vi "Perform measurements.vi"(6 "Measurement configuration":T2={"Number of channels to measure"=0, "Full scale range"=10.0, "Analog source input channels"=[], "Analog source resource names"=[], "Frequency"=1000.0, "Amplitude"=-1.0, "Digital capture resource name"="", "Digital capture sample rate"=800000.0, "Digital capture samples"=800000}, 10 "DPI Session":refnum<k15>, 11 "DPI Bitfile reference":refnum<k20>) -> (0 "error out":errorcluster, 2 "Measurement results":T1)   [LabVIEW 2021, in "adc_acMultiChannelMeasurement.lvlib"]
uses:
  adc_acMultiChannelMeasurement.lvlib
  Measurement Configuration.ctl
  Measurement Results.ctl
  <vilib>/Utility/error.llb/Error Cluster From Error Code.vi
  <vilib>/rvi/errors/niLvFpgaAdjustHostInterfaceError.vi
  <instrlib>/niDigital/niDigital.llb/niDigital Burst Pattern (Burst Only).vi
  <vilib>/rvi/interface/nirviReadWriteControl/nirviReadWriteControl.xnode
  NiFpgaLv.dll
  <vilib>/rvi/interface/Simulation/niFpgaSimulationCallBeginRW.vi
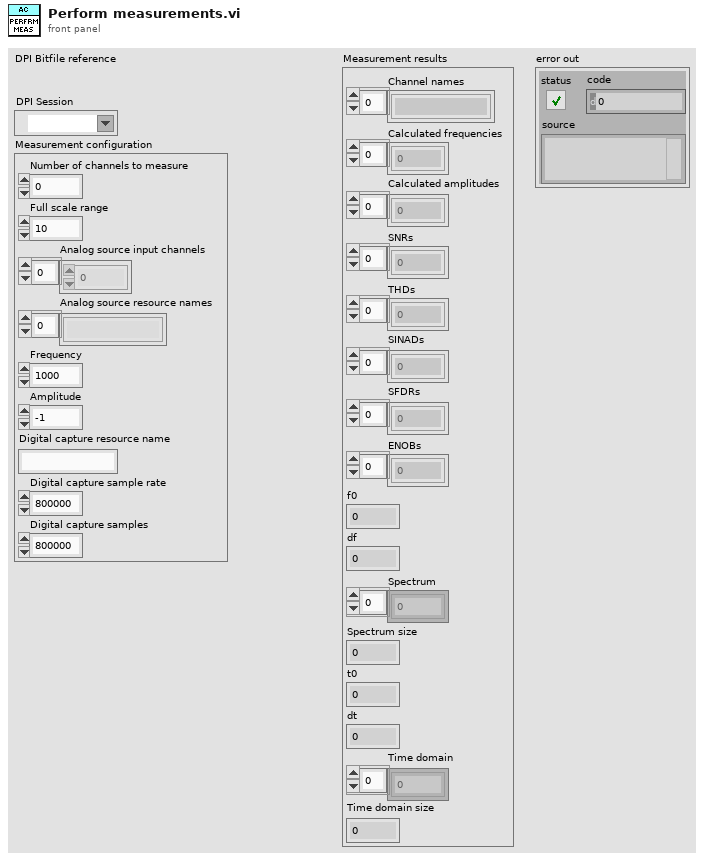
[diagram p1: front panel]
types:
  T1 = typedef "adc_acMultiChannelMeasurement.lvlib/Measurement Results.ctl" = cluster{"Channel names":string[], "Calculated frequencies":dbl[], "Calculated amplitudes":dbl[], "SNRs":dbl[], "THDs":dbl[], "SINADs":dbl[], "SFDRs":dbl[], "ENOBs":dbl[], "f0":dbl, "df":dbl, "Spectrum":dbl[], "Spectrum size":i32, "t0":dbl, "dt":dbl, "Time domain":dbl[], "Time domain size":i32}
  T2 = typedef "adc_acMultiChannelMeasurement.lvlib/Measurement Configuration.ctl" = cluster{"Number of channels to measure":i32, "Full scale range":dbl, "Analog source input channels":i32[], "Analog source resource names":string[], "Frequency":dbl, "Amplitude":dbl, "Digital capture resource name":string, "Digital capture sample rate":dbl, "Digital capture samples":u32}
  T3 = cluster{"Detected frequency":dbl, "Detected amplitude":dbl, "SNR":dbl, "THD":dbl, "SINAD":dbl, "SFDR":dbl, "ENOB":dbl}
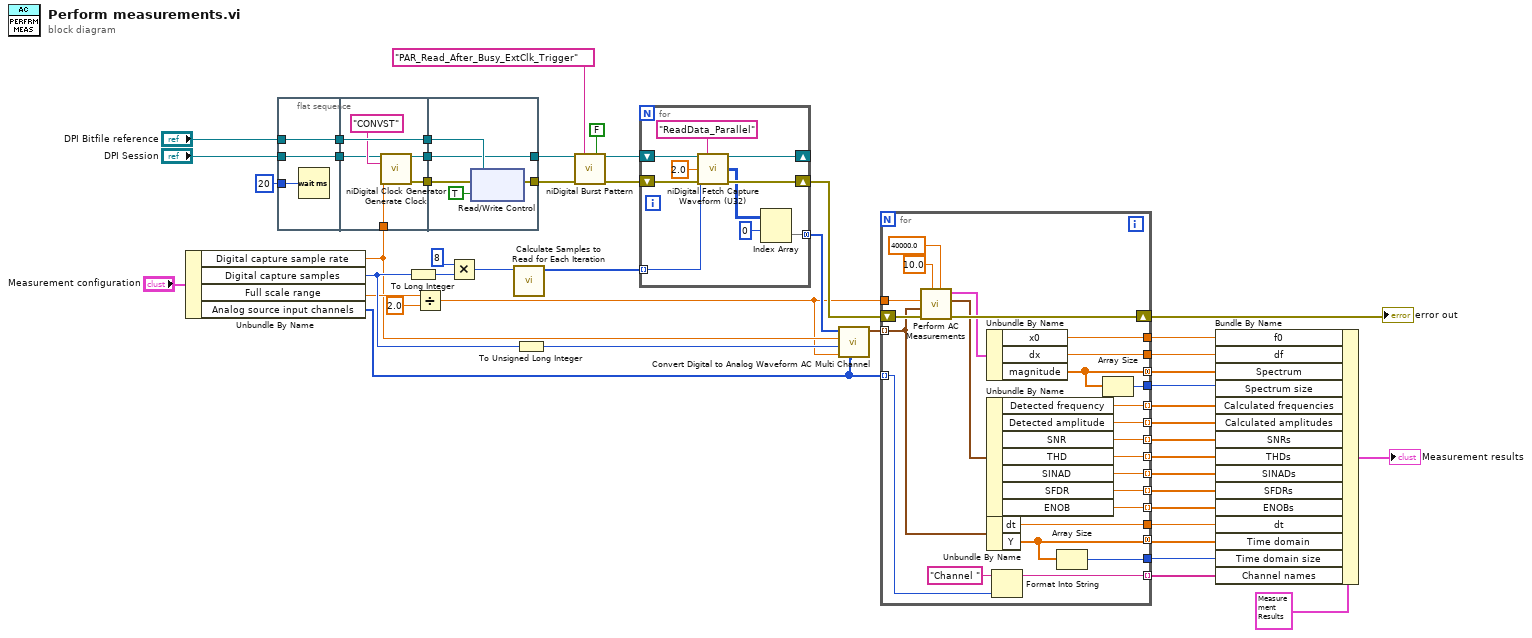
[diagram p0: block diagram]
diagram:
  n1 = Unbundle By Name("Measurement configuration") -> ("Digital capture sample rate"=w8:dbl, "Digital capture samples"=w13:u32, "Full scale range"=w10:dbl, "Analog source input channels"=w1:i32[])
  n2 = flat-sequence {
    tunnel: "DPI Session" -> [w49]
    tunnel: "DPI Bitfile reference" -> [w50]
    tunnel: [w50] -> w35
    tunnel: [w49] -> w34
    tunnel: u32 20 ("milliseconds to wait") -> [w48]
    tunnel: [w56] -> w33
    tunnel: [w54] -> w32
    tunnel: [w52] -> w31
    tunnel: w8 -> [w51]
    tunnel: w35 -> [w56]
    tunnel: w34 -> [w53]
    tunnel: [w61] -> w47
    tunnel: w33 -> [w60]
    tunnel: w32 -> [w58]
    tunnel: [w57] -> w36
    tunnel: w31 -> [w57]
    frame #0 {
      n3 = Wait (ms)(milliseconds to wait=w48) -> ()  [unwired: 1 out]
    }
    frame #1 {
      n4 = call <instrlib>:"niDigital Clock Generator Generate Clock.vi"("instrument handle"=w53, "channel list"="CONVST", "frequency (Hz)"=w51) -> ("instrument handle out"=w52:refnum<k15>, "error out"=w54:errorcluster)  [unwired: 11 in]
    }
    frame #2 {
      n5 = xnode "Read/Write Control"("FPGA VI Reference In"=w60, "error in"=w58, "active"=TRUE) -> ("error out"=w61:errorcluster)  [unwired: 1 out]
    }
  }
  n6 = To Long Integer(number=w13) -> (32bit integer=w12:i32)
  n7 = Divide(x=w10, y=2.0) -> (x/y=w6:dbl)
  n8 = Multiply(x=8 ("y"), y=w12) -> (x*y=w38:i32)
  n9 = call "Calculate Samples to Read for Each Iteration.vi"("total samples to read"=w38) -> ("samples to read"=w44:i32[])  [unwired: 10 in]
  n10 = To Unsigned Long Integer(number=w13) -> (unsigned 32bit integer=w7:u32)
  n11 = call-poly <instrlib>:"niDigital Burst Pattern.vi"("instrument handle"=w36, "start label"="PAR_Read_After_Busy_ExtClk_Trigger", "wait until done? (T)"=FALSE, "error in"=w47) -> ("instrument handle out"=w45:refnum<k15>, "error out"=w46:errorcluster)  [unwired: 10 in]
  n12 = for {
    tunnel: w44 -> [w62] mode=indexing
    shift-right: [w66] -> _
    shift-left: w45 -> [w71]
    shift-right: [w65] -> w29
    shift-left: w46 -> [w70]
    tunnel: [w67] -> w9 mode=concatenating
    n13 = call <instrlib>:"niDigital Fetch Capture Waveform (U32).vi"("instrument handle"=w71, "waveform name"="ReadData_Parallel", "timeout (s)"=2.0, "samples to read"=w62, "error in"=w70) -> ("instrument handle out"=w66:refnum<k15>, "data"=w63:u32[][], "error out"=w65:errorcluster)  [unwired: 8 in]
    n14 = Index Array(array=w63, index (row)=0) -> (element=w67:u32[])  [unwired: 1 in]
  }
  n15 = call "Convert Digital to Analog Waveform AC Multi Channel.vi"("Channels index"=w1, "full scale range"=w6, "Number of samples"=w7, "Sample rate"=w8, "Digital Waveform"=w9) -> ("Waveforms"=w5:waveform(dbl)[])  [unwired: 6 in]
  n16 = for {
    tunnel: [w91] -> w26
    tunnel: [w90] -> w25
    tunnel: [w76] -> w24 mode=concatenating
    tunnel: [w88] -> w23 mode=indexing
    tunnel: [w87] -> w22 mode=indexing
    tunnel: [w86] -> w21 mode=indexing
    tunnel: [w85] -> w20 mode=indexing
    tunnel: [w84] -> w19 mode=indexing
    tunnel: [w83] -> w18 mode=indexing
    tunnel: [w82] -> w17 mode=indexing
    tunnel: [w81] -> w16
    tunnel: [w78] -> w15 mode=concatenating
    tunnel: w6 -> [w80]
    shift-right: [w93] -> w28
    shift-left: w29 -> [w94]
    tunnel: w5 -> [w79] mode=indexing
    tunnel: [w77] -> w4
    tunnel: [w75] -> w3
    tunnel: [w73] -> w2 mode=indexing
    tunnel: w1 -> [w72] mode=indexing
    n17 = call "Perform AC Measurements.vi"("stop frequency"=40000.0, "start frequency"=10.0, "error in (no error)"=w94, "analog waveform"=w79, "input range (pk)"=w80) -> ("error out"=w93:errorcluster, "AC measurement results"=w89:T3, "frequency domain"=w92:cluster{"x0":dbl, "dx":dbl, "magnitude":dbl[]})  [unwired: 4 in]
    n18 = Unbundle By Name(w92) -> ("x0"=w91:dbl, "dx"=w90:dbl, "magnitude"=w76:dbl[])
    n19 = Unbundle By Name(w89) -> ("Detected frequency"=w88:dbl, "Detected amplitude"=w87:dbl, "SNR"=w86:dbl, "THD"=w85:dbl, "SINAD"=w84:dbl, "SFDR"=w83:dbl, "ENOB"=w82:dbl)
    n20 = Unbundle By Name(w79) -> ("dt"=w81:dbl, "Y"=w78:dbl[])
    n21 = Format Into String(initial string="Channel ", w72) -> (resulting string=w73:string)  [unwired: 2 in, 1 out]
    n22 = Array Size(array=w78) -> (size(s)=w77:i32)
    n23 = Array Size(array=w76) -> (size(s)=w75:i32)
  }
  "error out" <- w28
  n24 = Bundle By Name(cluster=T1 {"Channel names"=[], "Calculated frequencies"=[], "Calculated amplitudes"=[], "SNRs"=[], "THDs"=[], "SINADs"=[], "SFDRs"=[], "ENOBs"=[], "f0"=0.0, "df"=0.0, "Spectrum"=[], "Spectrum size"=0, "t0"=0.0, "dt"=0.0, "Time domain"=[], "Time domain size"=0} ("Measurement Results"), "f0"=w26, "df"=w25, "Spectrum"=w24, "Spectrum size"=w3, "Calculated frequencies"=w23, "Calculated amplitudes"=w22, "SNRs"=w21, "THDs"=w20, "SINADs"=w19, "SFDRs"=w18, "ENOBs"=w17, "dt"=w16, "Time domain"=w15, "Time domain size"=w4, "Channel names"=w2) -> (→"Measurement results":T1)
